vi "BuildModule-Modified (SubVI).vi"(0 "Module width[mm]":dbl=97.54, 1 "Module Centre [mm]":cluster{"X":dbl, "Y":dbl, "Z":dbl}, 2 "Angle":dbl, 3 "Units":enum16{"mrad", "Radians", "Degrees"}(ring), 5 "Module height [mm]":dbl=97.54, 7 "x to fiducial [um]":dbl=230.0, 9 "y to fiducial [um]":dbl=1030.0, 11 "error in (no error)":errorcluster) -> (4 "Generated List of Module Coordinates":dbl[][](array[numeric]), 15 "error out":errorcluster)   [LabVIEW 2016]
panel:
  in  "Tab Control":T1(tab)
  out "lh [mm]":dbl
  out "lv [mm]":dbl
  out "A [mm]":cluster{"X":dbl, "Y":dbl, "Z":dbl}
  out "D [mm]":cluster{"X":dbl, "Y":dbl, "Z":dbl}
  out "B [mm]":cluster{"X":dbl, "Y":dbl, "Z":dbl}
  out "C [mm]":cluster{"X":dbl, "Y":dbl, "Z":dbl}
  out "A-B coordinates":cluster{"X":dbl, "Y":dbl, "Z":dbl}
  out "Length":dbl
  out "x, centre":dbl
  out "y, centre":dbl
  out "X interfid distance (should match length)":dbl
  out "Y interfid distance (should match height)":dbl
  out "Created Module Graph":cluster{dbl[], dbl[]}(graph)
  # "PLAN VIRTUAL STAVE: BuildModule Brandeis University - Brookhaven National Laboratory * ATLAS Phase II Inner Tracker Upgrade"
  # "This SubVI takes a centre coordinate and computes the positions of modules associated with that centre.\nThe SubVI also accepts a rotation angle to pivot the module."
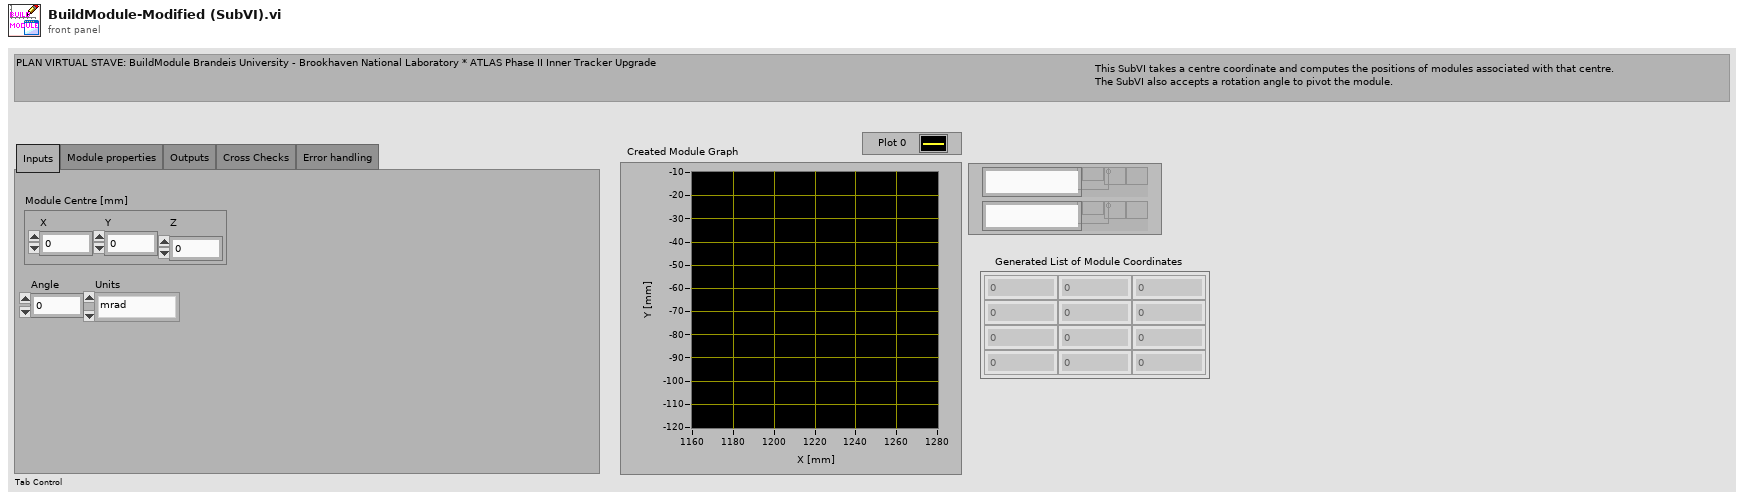
[diagram p1: front panel]
types:
  T1 = enum32{"Inputs", "Module properties", "Outputs", "Cross Checks", "Error handling"}
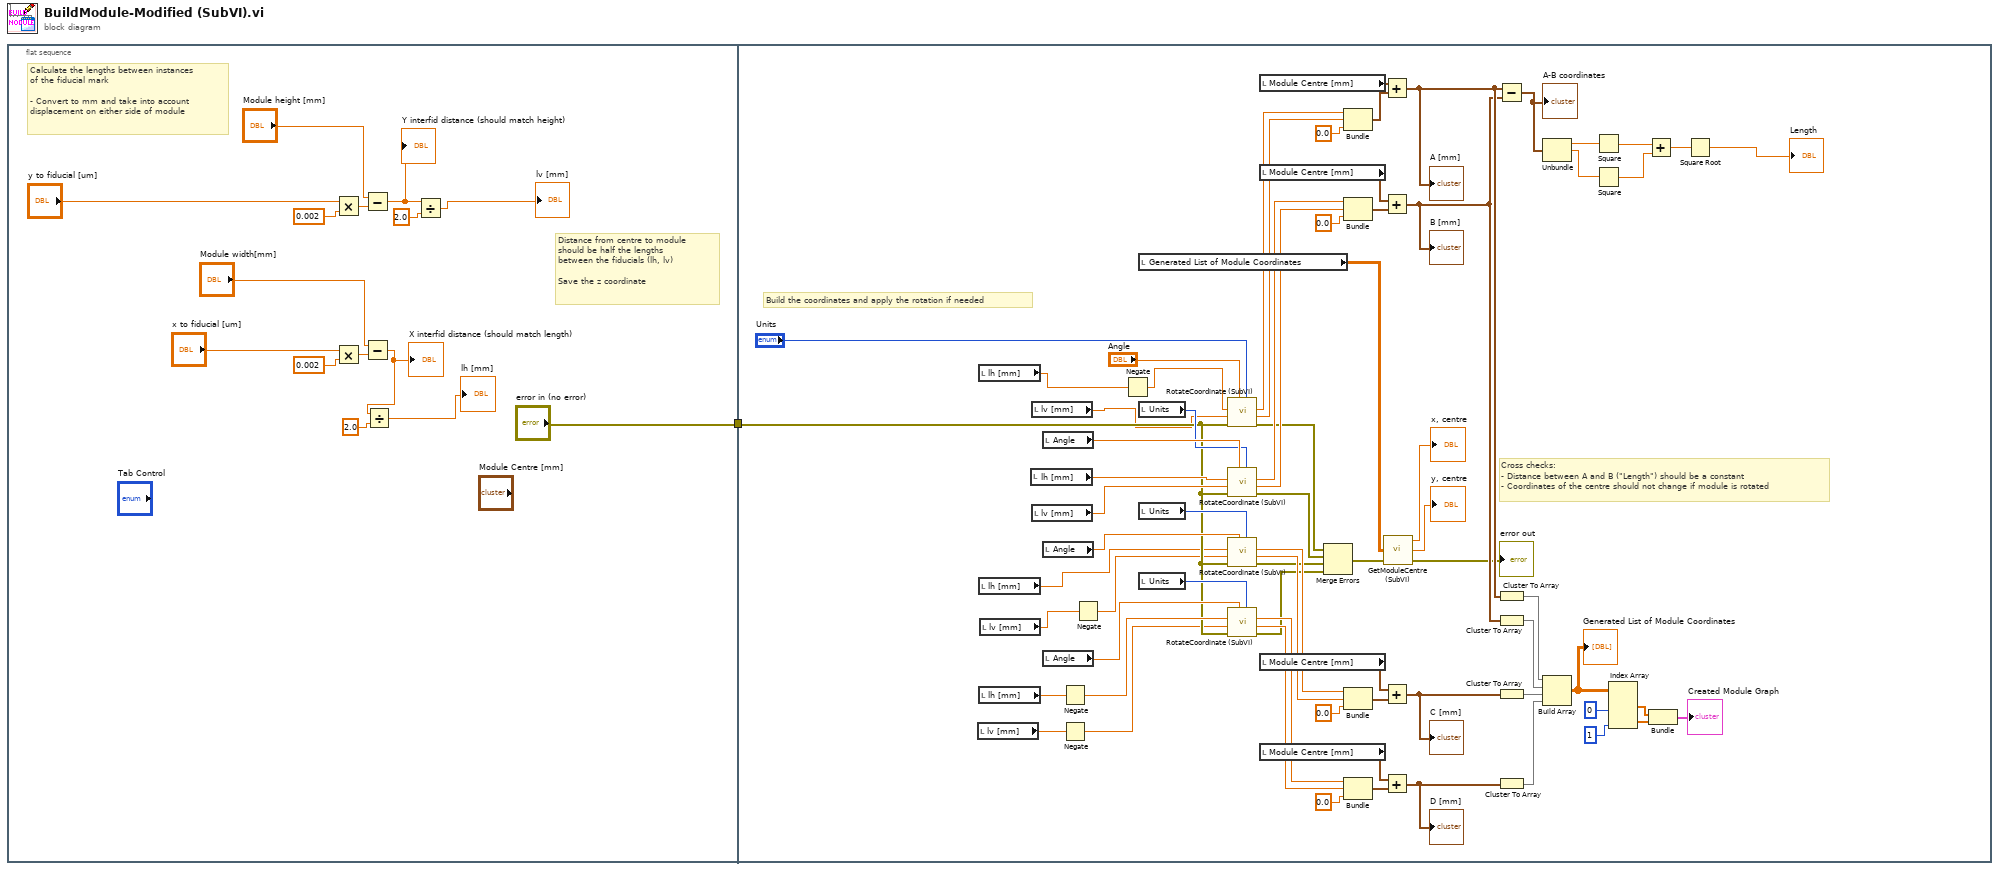
[diagram p0: block diagram]
diagram:
  n1 = flat-sequence {
    tunnel: ["error in (no error)"] -> w1
    tunnel: w1 -> [w35]
    frame #0 {
      # "Calculate the lengths between instances\nof the fiducial mark\n\n- Convert to mm and take into account\ndisplacement on either side of module"
      # "Distance from centre to module \nshould be half the lengths\nbetween the fiducials (lh, lv)\n\nSave the z coordinate"
      n2 = Multiply(x="y to fiducial [um]", y=0.002) -> (x*y=w8:dbl)
      n3 = Multiply(x="x to fiducial [um]", y=0.002) -> (x*y=w10:dbl)
      n4 = Subtract(x="Module height [mm]", y=w8) -> (x-y=w3:dbl)
      "Y interfid distance (should match height)" <- w3
      n5 = Subtract(x="Module width[mm]", y=w10) -> (x-y=w5:dbl)
      "X interfid distance (should match length)" <- w5
      n6 = Divide(x=w5, y=2.0) -> (x/y=→"lh [mm]":dbl)
      n7 = Divide(x=w3, y=2.0) -> (x/y=→"lv [mm]":dbl)
    }
    frame #1 {
      # "Build the coordinates and apply the rotation if needed"
      # "Cross checks: \n- Distance between A and B (\"Length\") should be a constant\n- Coordinates of the centre should not change if module is rotated"
      n8 = local read "lv [mm]"() -> (w24:dbl)
      n9 = local read "lh [mm]"() -> (w21:dbl)
      n10 = local read "lh [mm]"() -> (w19:dbl)
      n11 = local read "lh [mm]"() -> (w62:dbl)
      n12 = local read "lv [mm]"() -> (w18:dbl)
      n13 = local read "lh [mm]"() -> (w41:dbl)
      n14 = local read "lv [mm]"() -> (w22:dbl)
      n15 = local read "lv [mm]"() -> (w64:dbl)
      n16 = local read "Angle"() -> (w68:dbl)
      n17 = local read "Angle"() -> (w69:dbl)
      n18 = local read "Angle"() -> (w63:dbl)
      n19 = Negate(x=w62) -> (-x=w40:dbl)
      n20 = Negate(x=w24) -> (-x=w23:dbl)
      n21 = Negate(x=w18) -> (-x=w17:dbl)
      n22 = Negate(x=w21) -> (-x=w20:dbl)
      n23 = local read "Generated List of Module Coordinates"() -> (w83:dbl[][])
      n24 = local read "Units"() -> (w67:enum16{"mrad", "Radians", "Degrees"})
      n25 = local read "Units"() -> (w70:enum16{"mrad", "Radians", "Degrees"})
      n26 = local read "Units"() -> (w71:enum16{"mrad", "Radians", "Degrees"})
      n27 = call "RotateCoordinate (SubVI).vi"("Units"="Units", "Angle"="Angle", "error in (no error)"=w35, "y"=w22, "x"=w20) -> ("error out"=w34:errorcluster, "y'"=w44:dbl, "x'"=w45:dbl)  [unwired: 4 in]
      n28 = call "RotateCoordinate (SubVI).vi"("Units"=w67, "Angle"=w68, "error in (no error)"=w35, "y"=w64, "x"=w41) -> ("error out"=w33:errorcluster, "y'"=w42:dbl, "x'"=w43:dbl)  [unwired: 4 in]
      n29 = call "RotateCoordinate (SubVI).vi"("Units"=w70, "Angle"=w69, "error in (no error)"=w35, "y"=w17, "x"=w19) -> ("error out"=w32:errorcluster, "y'"=w48:dbl, "x'"=w49:dbl)  [unwired: 4 in]
      n30 = call "RotateCoordinate (SubVI).vi"("Units"=w71, "Angle"=w63, "error in (no error)"=w35, "y"=w23, "x"=w40) -> ("error out"=w31:errorcluster, "y'"=w38:dbl, "x'"=w39:dbl)  [unwired: 4 in]
      n31 = local read "Module Centre [mm]"() -> (w54:cluster{"X":dbl, "Y":dbl, "Z":dbl})
      n32 = local read "Module Centre [mm]"() -> (w59:cluster{"X":dbl, "Y":dbl, "Z":dbl})
      n33 = local read "Module Centre [mm]"() -> (w58:cluster{"X":dbl, "Y":dbl, "Z":dbl})
      n34 = local read "Module Centre [mm]"() -> (w56:cluster{"X":dbl, "Y":dbl, "Z":dbl})
      n35 = Merge Errors(w34, w33, w32, w31) -> (w80:errorcluster)
      n36 = Bundle("x'"=w45, "y'"=w44, "y"=0.0) -> (w46:cluster{"x'":dbl, "y'":dbl, "y":dbl})  [unwired: 1 in]
      n37 = Bundle("x'"=w43, "y'"=w42, "y"=0.0) -> (w36:cluster{"x'":dbl, "y'":dbl, "y":dbl})  [unwired: 1 in]
      n38 = Bundle("x'"=w49, "y'"=w48, "y"=0.0) -> (w47:cluster{"x'":dbl, "y'":dbl, "y":dbl})  [unwired: 1 in]
      n39 = Bundle("x'"=w39, "y'"=w38, "y"=0.0) -> (w37:cluster{"x'":dbl, "y'":dbl, "y":dbl})  [unwired: 1 in]
      n40 = Add(x=w54, y=w46) -> (x+y=w30:cluster{dbl, dbl, dbl})
      "A [mm]" <- w30
      n41 = Add(x=w59, y=w36) -> (x+y=w29:cluster{dbl, dbl, dbl})
      "B [mm]" <- w29
      n42 = Add(x=w58, y=w47) -> (x+y=w57:cluster{dbl, dbl, dbl})
      "C [mm]" <- w57
      n43 = Add(x=w56, y=w37) -> (x+y=w55:cluster{dbl, dbl, dbl})
      "D [mm]" <- w55
      n44 = call "GetModuleCentre (SubVI).vi"("error in (no error)"=w80, "4x3 Array of Fiducial Coordinates"=w83) -> ("error out"=→"error out":errorcluster, "y, centre"=→"y, centre":dbl, "x, centre"=→"x, centre":dbl)  [unwired: 1 in]
      n45 = Subtract(x=w30, y=w29) -> (x-y=w27:cluster{dbl, dbl, dbl})
      "A-B coordinates" <- w27
      n46 = Cluster To Array(cluster=w30) -> (array=w72:dbl[])
      n47 = Cluster To Array(cluster=w29) -> (array=w73:dbl[])
      n48 = Cluster To Array(cluster=w57) -> (array=w74:dbl[])
      n49 = Cluster To Array(cluster=w55) -> (array=w75:dbl[])
      n50 = Unbundle(w27) -> (w26:dbl, w25:dbl)  [unwired: 1 out]
      n51 = Build Array(w72, w73, w74, w75) -> (w61:dbl[][])
      "Generated List of Module Coordinates" <- w61
      n52 = Square(x=w26) -> (x^2=w87:dbl)
      n53 = Square(x=w25) -> (x^2=w86:dbl)
      n54 = Index Array(array=w61, index (col) #1=0 ("disabled index (col)"), index (col) #2=1 ("index (col)")) -> (element #1=w78:dbl[], element #2=w79:dbl[])  [unwired: 2 in]
      n55 = Add(x=w87, y=w86) -> (x+y=w85:dbl)
      n56 = Bundle(w78, w79) -> (→"Created Module Graph":cluster{dbl[], dbl[]})  [unwired: 1 in]
      n57 = Square Root(x=w85) -> (sqrt(x)=→"Length":dbl)
    }
  }
